vi "testCreateEnumArray.vi"(8 "error in (no error)":errorcluster) -> (0 "error out":errorcluster)   [LabVIEW 2018]
uses:
  SALTypeGenerator/Elements/Enum/Enum.lvclass
  SALTypeGenerator/Elements/Enum/Enum.lvclass/Enum.ctl
  <vilib>/addons/_JKI Toolkits/Caraya/classes/Assert/Assert Equal Value_Variant.vi
  <vilib>/addons/_JKI Toolkits/Caraya/classes/Test/Test.lvclass
  <vilib>/addons/_JKI Toolkits/Caraya/classes/Assert/Assert.lvclass
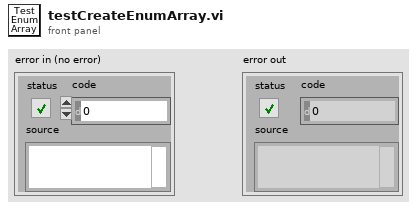
[diagram p1: front panel]
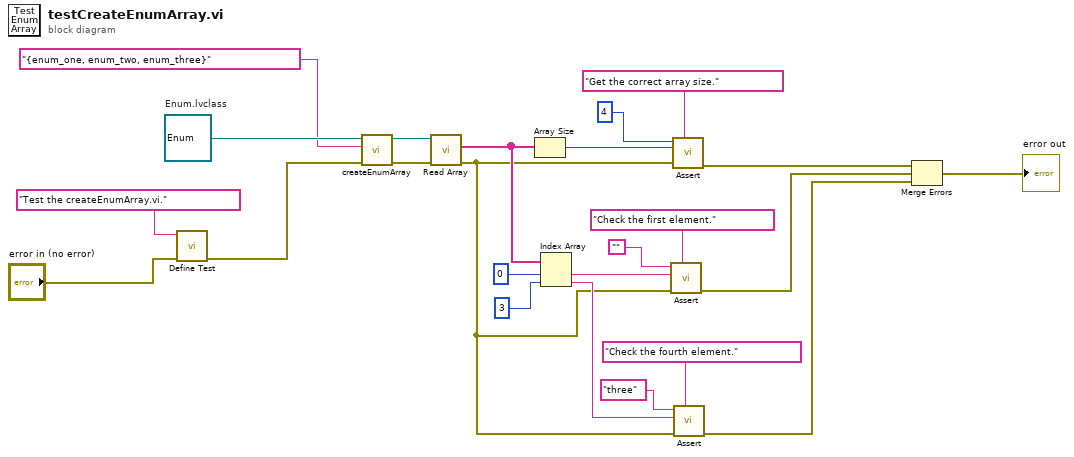
[diagram p0: block diagram]
diagram:
  w24 = refnum<class "Enum.lvclass"> refnum  # Enum.lvclass
  n1 = call <vilib>:"Define Test.vi"("error in (no error)"="error in (no error)", "Label (VI Title)"="Test the createEnumArray.vi.") -> ("error out"=w18:errorcluster)  [unwired: 9 in]
  n2 = call "createEnumArray.vi"("error in (no error)"=w18, "enums"="{enum_one, enum_two, enum_three}", "Enum in"=w24) -> ("error out"=w22:errorcluster, "Enum out"=w23:refnum<class "Enum.lvclass">)  [unwired: 7 in]
  n3 = call "Read Array.vi"("error in (no error)"=w22, "Enum in"=w23) -> ("error out"=w9:errorcluster, "Array"=w14:string[])  [unwired: 7 in, 1 out]
  n4 = Array Size(array=w14) -> (size(s)=w17:i32)
  n5 = Index Array(array=w14, index #1=0 ("index"), index #2=3 ("index")) -> (element #1=w11:string, element #2=w10:string)
  n6 = call-poly <vilib>:"Assert.vi"("Label"="Check the first element.", "error in (no error)"=w9, "Y"=w11, "X"="") -> ("error out"=w3:errorcluster)  [unwired: 7 in]
  n7 = call-poly <vilib>:"Assert.vi"("Label"="Get the correct array size.", "error in (no error)"=w9, "Y"=w17, "X"=4) -> ("error out"=w4:errorcluster)  [unwired: 7 in]
  n8 = call-poly <vilib>:"Assert.vi"("Label"="Check the fourth element.", "error in (no error)"=w9, "Y"=w10, "X"="three") -> ("error out"=w2:errorcluster)  [unwired: 7 in]
  n9 = Merge Errors(w4, w3, w2) -> (→"error out":errorcluster)
